vi "Contains.vi"(10 "Item":string, 11 "List":string[](array[string])) -> (2 "Contains":bool)   [LabVIEW 2017, in "MessageGen.lvlib"]
uses:
  <vilib>/addons/InsightCM/MessageBus/CodeGen/MessageGen.lvlib
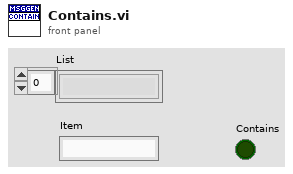
[diagram p1: front panel]
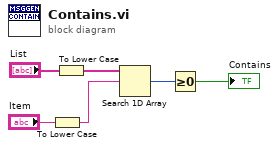
[diagram p0: block diagram]
diagram:
  n1 = To Lower Case(string="Item") -> (all lower case string=w1:string)
  n2 = To Lower Case(string="List") -> (all lower case string=w2:string[])
  n3 = Search 1D Array(1D array=w2, element=w1) -> (index of element=w4:i32)  [unwired: 1 in]
  n4 = Greater Or Equal To 0?(x=w4) -> (x >= 0?=→"Contains":bool)
